vi "Reflux BatchD.vi"() -> ()   [LabVIEW 2017]
panel:
  in  "Reflux Ratio":dbl
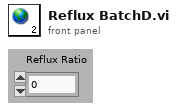
[diagram p1: front panel]
diagram:
